vi "Show Data Logger.vi"(8 "error in":errorcluster, 11 "Study Actor in":refnum<class "Study Actor.lvclass">) -> (0 "error out":errorcluster, 3 "Study Actor out":refnum<class "Study Actor.lvclass">)   [LabVIEW 2024, in "Study Actor.lvlib" / "Study Actor.lvclass"]
uses:
  Study Actor.lvclass
  Study Actor.lvclass/Study Actor.ctl
  <vilib>/ActorFramework/Message Enqueuer/Message Enqueuer.lvclass/Message Enqueuer.ctl
  <vilib>/ActorFramework/Message Enqueuer/Enqueue.vi
  Series/ISeries Actor/ISeries Actor Messages/Show Data Logger Msg/Show Data Logger Msg.lvclass
  <vilib>/Utility/LVClass/Get LV Class Name.vi
  <resource>/AFDebug/Generate Trace for Message.vi
  <vilib>/ActorFramework/Message Priority Queue/Priority Enqueue.vi
  <vilib>/ActorFramework/Message Enqueuer/Message Enqueuer.lvclass
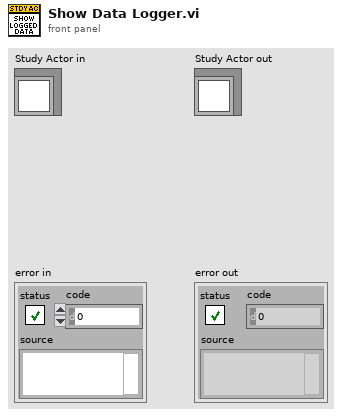
[diagram p1: front panel]
types:
  T1 = map{string, refnum<class "Message Enqueuer.lvclass">}
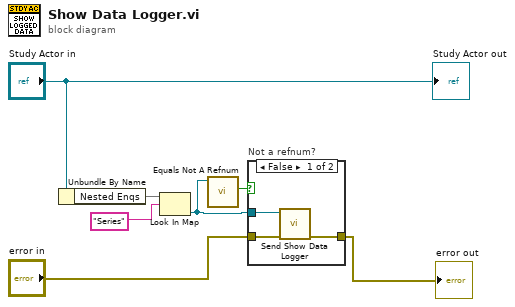
[diagram p0: block diagram]
diagram:
  n1 = Unbundle By Name("Study Actor in") -> ("Nested Enqs"=w6:T1)
  n2 = Look In Map(map=w6, key="Series") -> (value=w1:refnum<class "Message Enqueuer.lvclass">)  [unwired: 1 in, 1 out]
  n3 = call <vilib>:"Equals Not A Refnum.vi"("Message Enqueuer"=w1) -> ("Not a refnum?"=w2:bool)  [unwired: 10 in]
  n4 = case "Not a refnum?" shown="False" w2 {
    tunnel: w1 -> [w10 _]
    tunnel: "error in" -> [w9 w11]
    tunnel: [w8 w11] -> w3
    frame False {
      n5 = call "Send Show Data Logger.vi"("error in (no error)"=w9, "Message Enqueuer"=w10) -> ("error out"=w8:errorcluster)  [unwired: 8 in, 1 out]
    }
    frame True {
    }
  }
  "error out" <- w3
  "Study Actor out" <- "Study Actor in"
